vi "Untitled 5.vi"() -> ()   [LabVIEW 2014]
panel:
  out "output variable":dbl
  out "x-y":u32
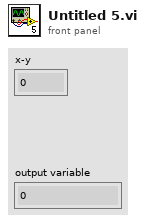
[diagram p1: front panel]
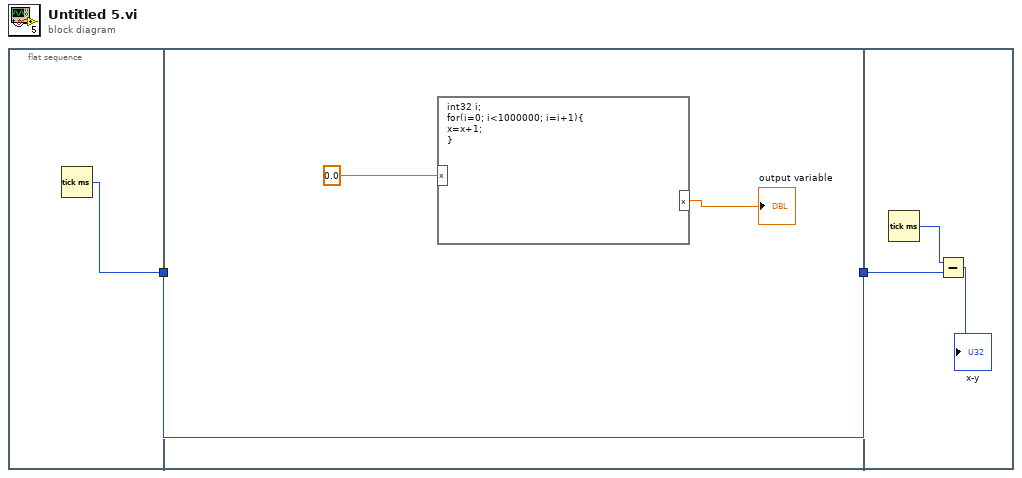
[diagram p0: block diagram]
diagram:
  n1 = flat-sequence {
    tunnel: [w3] -> w2
    tunnel: w2 -> [w6]
    tunnel: [w6] -> w1
    tunnel: w1 -> [w8]
    frame #0 {
      n2 = Tick Count (ms)() -> (millisecond timer value=w3:u32)
    }
    frame #1 {
      n3 = formula code="int32 i;\nfor(i=0; i<1000000; i=i+1){\nx=x+1;\n}"("x"=0.0 ("input variable")) -> ("x"=→"output variable":dbl)
    }
    frame #2 {
      n4 = Tick Count (ms)() -> (millisecond timer value=w9:u32)
      n5 = Subtract(x=w9, y=w8) -> (x-y=→"x-y":u32)
    }
  }
